vi "Get File Attributes.vi"(6 "timeout (ms)":i32=30000, 8 "error in":errorcluster, 10 "remote path":string, 11 "session in":refnum<class "Session.lvclass">) -> (0 "error out":errorcluster, 2 "file attributes":refnum<class "File Attributes.lvclass">, 3 "session out":refnum<class "Session.lvclass">)   [LabVIEW 2020, in "NI_SFTP.lvlib"]
doc: "Returns information about a remote file or directory."
uses:
  <vilib>/net/SFTP/NI_SFTP.lvlib
  <vilib>/net/SFTP/Session/Session.lvclass
  <vilib>/net/SFTP/File Attributes/File Attributes.lvclass
  <vilib>/net/SFTP/File Attributes/File Attributes.lvclass/File Attributes.ctl
  <vilib>/Utility/Deadline/NI_Deadline.lvlib
  <vilib>/net/SFTP/API/Support/Command/SSH_FXP_STAT/SSH_FXP_STAT.lvclass
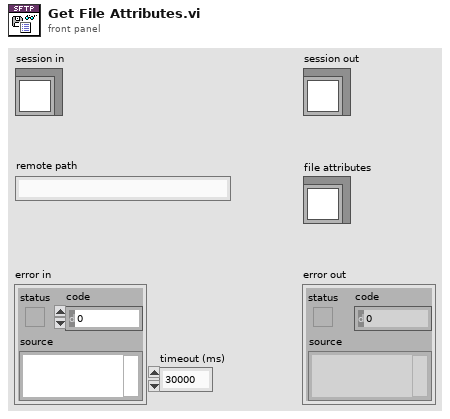
[diagram p1: front panel]
types:
  T1 = typedef "NI_Deadline.lvlib/Deadline.ctl" = cluster{"mode":T2, "deadline (ms)":u32}
  T2 = typedef "NI_Deadline.lvlib/Mode.ctl" = enum16{"Relative", "Use deadline", "Wait forever", "Nonblocking", "N/A"}
  T3 = typedef "NI_SFTP.lvlib/File Attributes.ctl" = cluster{"SSH_FILEXFER_ATTR_SIZE":bool, "size":u64, "SSH_FILEXFER_ATTR_UIDGID":bool, "uid":u32, "gid":u32, "SSH_FILEXFER_ATTR_PERMISSIONS":bool, "permissions":u32, "SSH_FILEXFER_ATTR_ACMODTIME":bool, "atime":u32, "mtime":u32, "extended":map{string, string}}
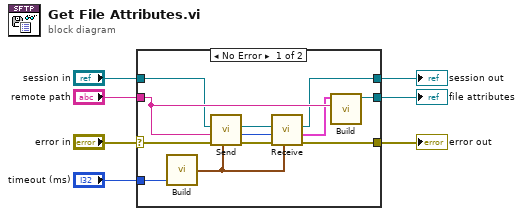
[diagram p0: block diagram]
diagram:
  n1 = case shown="No Error" "error in" {
    selector: "error in" -> [w18 w21]
    tunnel: [w17 w21] -> w5
    tunnel: [w8 w20] -> w3
    tunnel: "session in" -> [w11 w20]
    tunnel: "timeout (ms)" -> [w16 _]
    tunnel: "remote path" -> [w12 _]
    tunnel: [w13 _] -> w1
    frame No Error {
      n2 = call <vilib>:"Build.vi"("timeout (ms)"=w16) -> ("Deadline out"=w15:T1)  [unwired: 2 in]
      n3 = call <vilib>:"Send.vi"("deadline"=w15, "error in (no error)"=w18, "path"=w12, "session in"=w11) -> ("error out"=w19:errorcluster, "request id"=w10:u32, "session out"=w14:refnum<class "Session.lvclass">)  [unwired: 4 in, 1 out]
      n4 = call <vilib>:"Receive.vi"("deadline"=w15, "error in (no error)"=w19, "request id"=w10, "session in"=w14) -> ("error out"=w17:errorcluster, "file attributes"=w9:T3, "session out"=w8:refnum<class "Session.lvclass">)  [unwired: 4 in, 1 out]
      n5 = call <vilib>:"Build.vi"("file name"=w12, "file attributes"=w9) -> ("file attributes out"=w13:refnum<class "File Attributes.lvclass">)  [unwired: 9 in]
    }
    frame Error {
    }
  }
  "error out" <- w5
  "session out" <- w3
  "file attributes" <- w1
